vi "Stop Measurements Command.vi"(8 "error in (no error)":errorcluster, 10 "Measurement Controller":string, 11 "Monitor-Pulse in":refnum<class "Monitor-Pulse.lvclass">) -> (0 "error out":errorcluster, 3 "Monitor-Pulse out":refnum<class "Monitor-Pulse.lvclass">)   [LabVIEW 2015, in "Monitor-Pulse.lvclass"]
uses:
  Monitor-Pulse.lvclass
  <vilib>/ActorFramework/Message Enqueuer/Message Enqueuer.lvclass/Message Enqueuer.ctl
  <vilib>/ActorFramework/Message Enqueuer/Enqueue.vi
  <vilib>/ActorFramework/Message Priority Queue/Priority Enqueue.vi
  Measure_core/Measure Controller Messages/Stop Measurements Msg/Stop Measurements Msg.lvclass
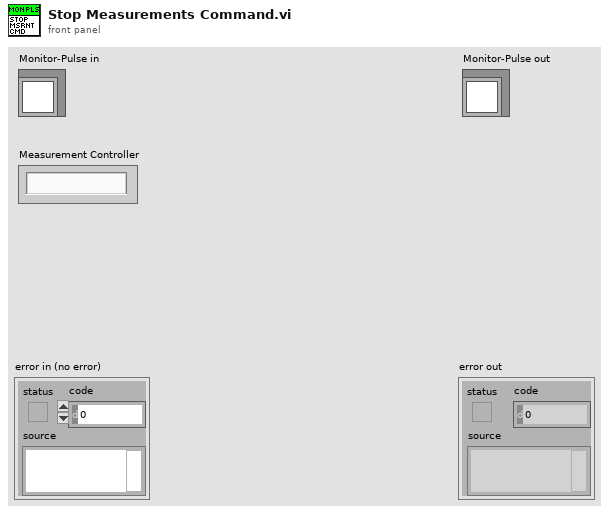
[diagram p1: front panel]
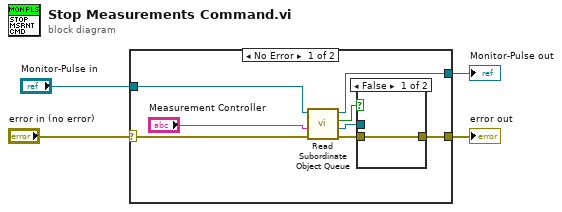
[diagram p0: block diagram]
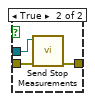
[diagram p2: hidden frame]
diagram:
  n1 = case shown="No Error" "error in (no error)" {
    selector: "error in (no error)" -> [w7 w18]
    tunnel: [w5 w18] -> w3
    tunnel: [w9 w17] -> w1
    tunnel: "Monitor-Pulse in" -> [w10 w17]
    frame No Error {
      n2 = call-dynamic "Read Subordinate Object Queue.vi"("error in (no error)"=w7, "Name"="Measurement Controller", "Measure Object in"=w10) -> ("error out"=w6:errorcluster, "Object Enqueuer"=w11:refnum<class "Message Enqueuer.lvclass">, "Found?"=w8:bool, "Measure Object out"=w9:refnum<class "Monitor-Pulse.lvclass">)  [unwired: 5 in]
      n3 = case shown="False" w8 {
        tunnel: w11 -> [_ w16]
        tunnel: w6 -> [w13 w15]
        tunnel: [w13 w14] -> w5
        frame False {
        }
        frame True {
          n4 = call "Send Stop Measurements.vi"("error in (no error)"=w15, "Message Enqueuer"=w16) -> ("error out"=w14:errorcluster)  [unwired: 8 in, 1 out]
        }
      }
    }
    frame Error {
    }
  }
  "error out" <- w3
  "Monitor-Pulse out" <- w1
